vi "Read Thermocouple Module.vi"(8 "error in":errorcluster, 11 "module in":refnum<class "Module.lvclass">) -> (0 "error out":errorcluster, 2 "channel settings":T1[](array[typedef]), 3 "module out":refnum<class "Module.lvclass">)   [LabVIEW 2017, in "Scan Engine Scripting.lvlib" / "Module.lvclass"]
doc: "Returns the channel settings for a thermocouple module."
uses:
  Module.lvclass
  Mode Classes/Controls/thermocouple channel settings.ctl
  Channel Classes/Thermocouple Channel/Thermocouple Type.ctl
  Channel Classes/Thermocouple Channel/Measurement Units.ctl
  Mode Classes/Thermocouple Mode/Thermocouple Mode.lvclass
  Channel Classes/Thermocouple Channel/Thermocouple Channel.lvclass
  Scan Engine Scripting.lvlib
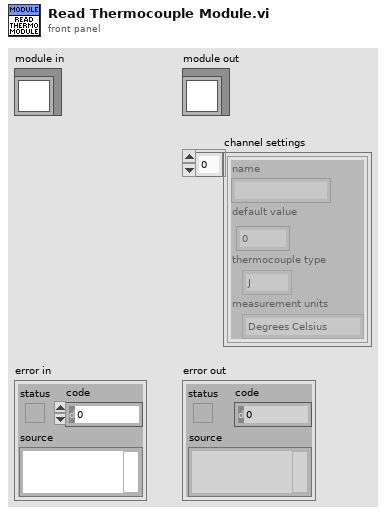
[diagram p1: front panel]
types:
  T1 = typedef "Scan Engine Scripting.lvlib/thermocouple channel settings.ctl" = cluster{"name":string, "default value":dbl, "thermocouple type":T2, "measurement units":T3}
  T2 = typedef "Scan Engine Scripting.lvlib/Thermocouple Channel.lvclass/Thermocouple Type.ctl" = enum16{"J", "K", "T", "E", "R", "S", "N", "B"}
  T3 = typedef "Scan Engine Scripting.lvlib/Thermocouple Channel.lvclass/Measurement Units.ctl" = enum16{"Raw Volts", "Degrees Kelvin", "Degrees Celsius", "Degrees Fahrenheit", "Degrees Rankine"}
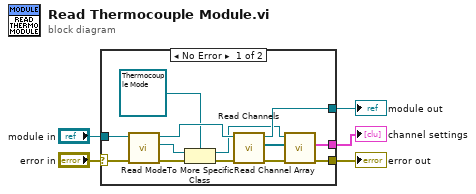
[diagram p0: block diagram]
diagram:
  n1 = case shown="No Error" "error in" {
    selector: "error in" -> [w17 w20]
    tunnel: [w6 w20] -> w2
    tunnel: [w13 w19] -> w3
    tunnel: "module in" -> [w18 w19]
    tunnel: [w7 _] -> w1
    frame No Error {
      n2 = call-dynamic "Read Mode.vi"("error in"=w17, "module in"=w18) -> ("error out"=w15:errorcluster, "mode"=w16:refnum<class "Mode.lvclass">, "module out"=w14:refnum<class "Module.lvclass">)  [unwired: 7 in]
      n3 = To More Specific Class(target class=refnum<class "Thermocouple Mode.lvclass"> refnum ("Scan Engine Scripting.lvlib:Analog Input Vrms Mode.lvclass"), reference=w16, error in=w15) -> (specific class reference=w9:refnum<class "Thermocouple Mode.lvclass">, error out=w11:errorcluster)
      n4 = call-dynamic "Read Channels.vi"("error in"=w11, "module in"=w14) -> ("error out"=w10:errorcluster, "channels"=w8:refnum<class "Channel.lvclass">[], "module out"=w13:refnum<class "Module.lvclass">)  [unwired: 7 in]
      n5 = call "Read Channel Array.vi"("error in"=w10, "channels"=w8, "thermocouple mode in"=w9) -> ("error out"=w6:errorcluster, "channel settings"=w7:T1[])  [unwired: 6 in, 1 out]
    }
    frame Error {
    }
  }
  "error out" <- w2
  "module out" <- w3
  "channel settings" <- w1
